vi "Init Subpanel UIs.vi"(8 "error in (no error)":errorcluster, 11 "BetterSearch in":refnum<class "BetterSearch.lvclass">) -> (0 "error out":errorcluster, 3 "BetterSearch out":refnum<class "BetterSearch.lvclass">)   [LabVIEW 2020, in "Better Search.lvlib" / "BetterSearch.lvclass"]
uses:
  BetterSearch.lvclass
  BetterSearch.lvclass/BetterSearch.ctl
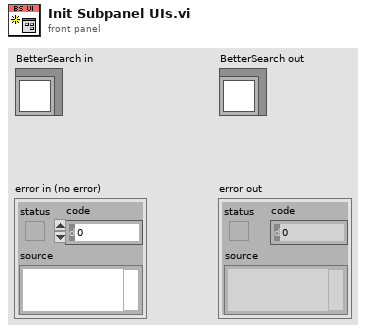
[diagram p1: front panel]
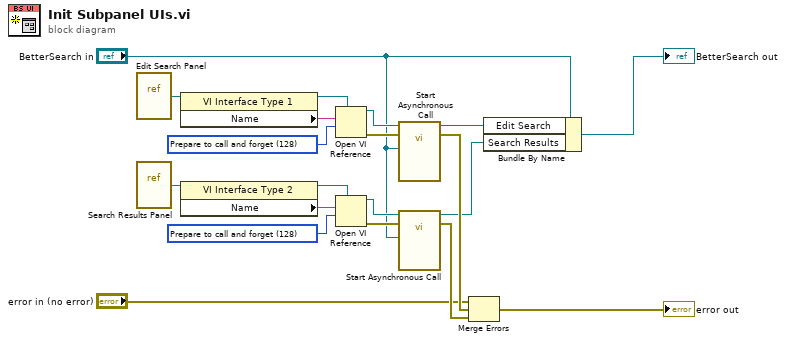
[diagram p0: block diagram]
diagram:
  w7 = 128 items=["Record modifications"=1, "Open templates for editing"=2, "Prompt user to save"=4, "Prepare for reentrant run"=8, "Prompt to find missing subVIs"=16, "Hide loading dialog box"=32, "Enable simultaneous calls"=64, "Prepare to call and forget"=128, "Simultaneous call and forget"=192, "Prepare to call and collect"=256, "Simultaneous call and collect"=320]
  w14 = 128 items=["Record modifications"=1, "Open templates for editing"=2, "Prompt user to save"=4, "Prepare for reentrant run"=8, "Prompt to find missing subVIs"=16, "Hide loading dialog box"=32, "Enable simultaneous calls"=64, "Prepare to call and forget"=128, "Simultaneous call and forget"=192, "Prepare to call and collect"=256, "Simultaneous call and collect"=320]
  n1 = vi-ref "Edit Search Panel.vi"() -> (w12:refnum<vi>)
  n2 = vi-ref "Search Results Panel.vi"() -> (w9:refnum<vi>)
  n3 = property class="VI Interface Type 1"(reference=w12) -> (reference out=w15:refnum<vi>, "Name"=w13:string)  [unwired: 1 in, 1 out]
  n4 = property class="VI Interface Type 2"(reference=w9) -> (reference out=w6:refnum<vi>, "Name"=w8:string)  [unwired: 1 in, 1 out]
  n5 = Open VI Reference(type specifier VI Refnum (for type only)=w15, vi path=w13, options=w14) -> (vi reference=w17:refnum<vi>, error out=w16:errorcluster)  [unwired: 3 in]
  n6 = Open VI Reference(type specifier VI Refnum (for type only)=w6, vi path=w8, options=w7) -> (vi reference=w4:refnum<vi>, error out=w5:errorcluster)  [unwired: 3 in]
  n7 = call-by-ref "Start Asynchronous Call"(reference=w17, error in=w16, "BetterSearch in"="BetterSearch in") -> (reference out=w10:refnum<vi>, error out=w19:errorcluster)  [unwired: 11 in]
  n8 = call-by-ref "Start Asynchronous Call"(reference=w4, error in=w5, "BetterSearch in"="BetterSearch in") -> (reference out=w2:refnum<vi>, error out=w20:errorcluster)  [unwired: 11 in]
  n9 = Merge Errors("error in (no error)", w19, w20) -> (→"error out":errorcluster)
  n10 = Bundle By Name(cluster="BetterSearch in", "Edit Search"=w10, "Search Results"=w2) -> (→"BetterSearch out":refnum<class "BetterSearch.lvclass">)
